vi "vector_v2.vi"() -> ()   [LabVIEW 2009]
panel:
  in  "stop":bool
  out "Vector LED-uri":bool[](array[boolean])=[TRUE, FALSE, TRUE, TRUE, FALSE, FALSE, FALSE, TRUE]
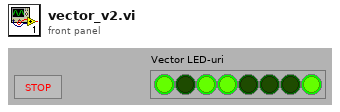
[diagram p1: front panel]
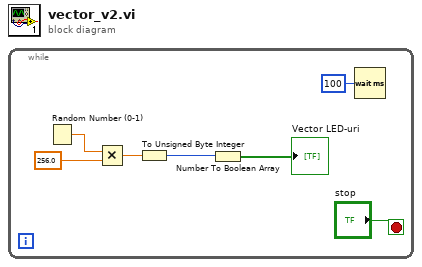
[diagram p0: block diagram]
diagram:
  n1 = while {
    stop <- "stop" stop-if-true
    n2 = Random Number (0-1)() -> (number: 0 to 1=w5:dbl)
    n3 = Multiply(x=w5, y=256.0) -> (x*y=w4:dbl)
    n4 = To Unsigned Byte Integer(number=w4) -> (unsigned 8bit integer=w6:u8)
    n5 = Number To Boolean Array(number=w6) -> (Boolean array=→"Vector LED-uri":bool[])
    n6 = Wait (ms)(milliseconds to wait=u32 100) -> ()  [unwired: 1 out]
  }
